vi "Test1_4.vi"() -> ()   [LabVIEW 2009]
uses:
  <instrlib>/Agilent 81150/Agilent 81150.lvlib
panel:
  in  "error in":errorcluster
  in  "Instrument VISA in":T1={"AWG VISA"="81160A", "Oscilloscope  VISA "="DSO80204B", "Integration Board IP"="172.16.7.43", "connection ID"=refnum}
  in  "Cycles Burst":i32=10000
  in  "DT_50_L0":i32[][](array[numeric])
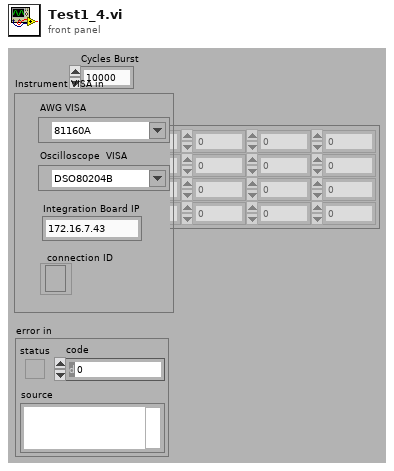
[diagram p1: front panel]
types:
  T1 = cluster{"AWG VISA":refnum<visa-resource-name>, "Oscilloscope  VISA ":refnum<visa-resource-name>, "Integration Board IP":string, "connection ID":refnum<k5>}
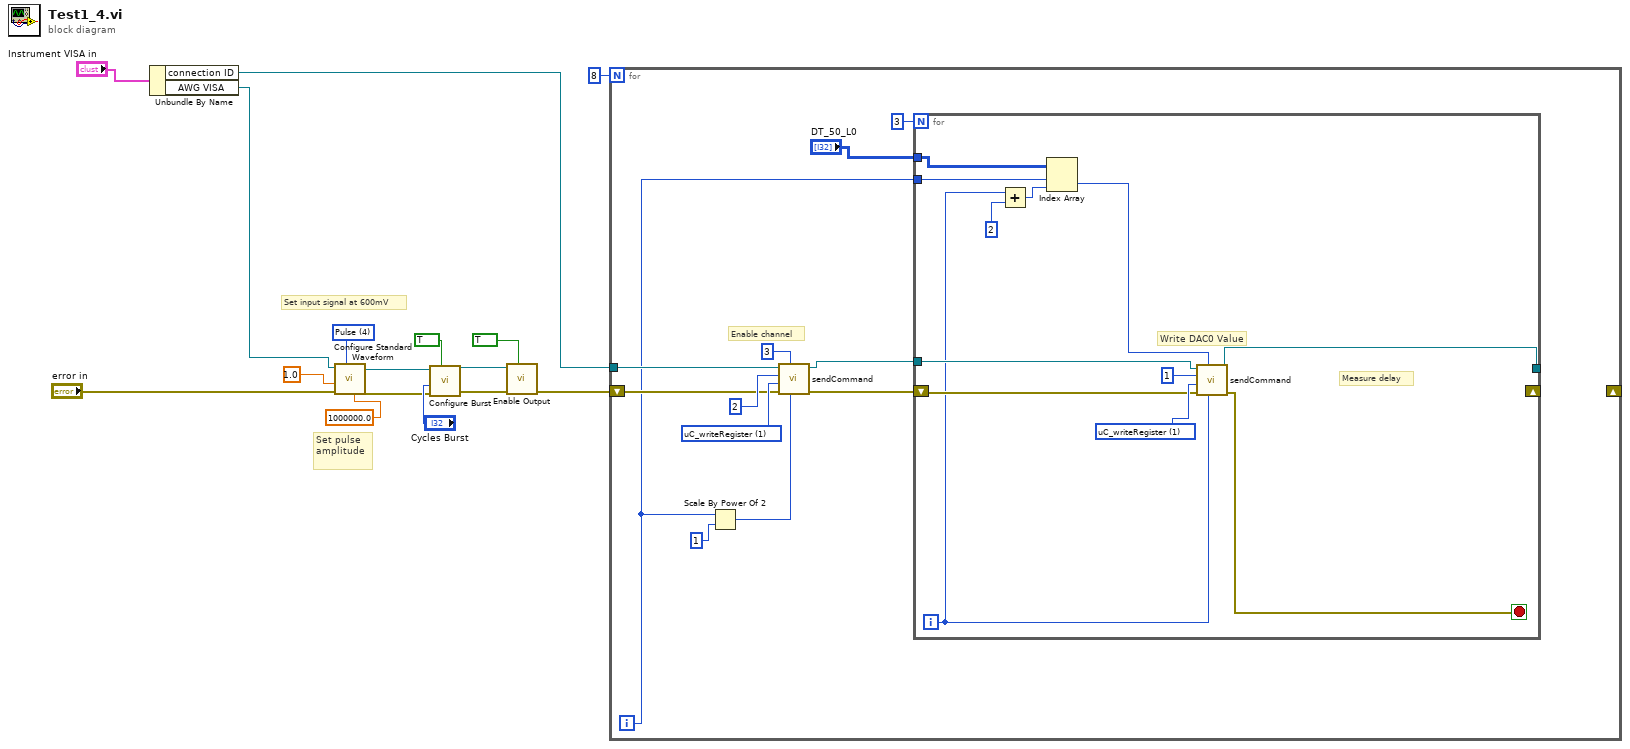
[diagram p0: block diagram]
diagram:
  w15 = u16 4 items=["Sine", "Square", "Ramp Up", "Ramp Down", "Pulse", "Noise", "DC"] ("Waveform (0: Sine)")
  # "Set input signal at 600mV"
  # "Set pulse amplitude"
  n1 = Unbundle By Name("Instrument VISA in") -> ("connection ID"=w3:refnum<k5>, "AWG VISA"=w1:refnum<visa-resource-name>)
  n2 = call <instrlib>:"Configure Standard Waveform.vi"("Frequency (1000.0 Hz)"=1000000.0, "Waveform (0: Sine)"=w15, "error in (no error)"="error in", "Amplitude (1.0 Vpp)"=1.0, "VISA resource name"=w1) -> ("error out"=w8:errorcluster, "VISA resource name out"=w7:refnum<visa-resource-name>)  [unwired: 5 in]
  n3 = call <instrlib>:"Configure Burst.vi"("Enable Burst (F: Disable)"=TRUE, "error in (no error)"=w8, "Burst Count (2)"="Cycles Burst", "VISA resource name"=w7) -> ("error out"=w11:errorcluster, "VISA resource name out"=w10:refnum<visa-resource-name>)  [unwired: 6 in]
  n4 = call <instrlib>:"Enable Output.vi"("Enable Output (T: Enable)"=TRUE, "error in (no error)"=w11, "VISA resource name"=w10) -> ("error out"=w2:errorcluster)  [unwired: 7 in, 1 out]
  n5 = for {
    N: 8 -> [_]
    tunnel: w3 -> [w20]
    shift-right: _ -> [_]
    shift-left: w2 -> [w19]
    i -> [w17]
    w26 = u16 1 items=["sendCommand"=9, "FPGA_writeRegister"=3, "FPGA_readRegister"=2, "uC_writeRegister"=1, "uC_readRegister"=0] ("Action")
    # "Enable channel"
    n6 = Scale By Power Of 2(n=w17, x=1) -> (x*2^n=w22:i32)
    n7 = call "sendCommand.vi"("Address"=w22, "Data"=3, "error in"=w19, "Action"=w26, "id_in"=2 ("id"), "connection ID"=w20) -> ("error out"=w21:errorcluster, "connection ID out"=w18:refnum<k5>)  [unwired: 1 in, 3 out]
    n8 = for {
      N: 3 -> [_]
      shift-right: _ -> [_]
      shift-left: w21 -> [w37]
      tunnel: "DT_50_L0" -> [w38]
      tunnel: [w35] -> _
      tunnel: w18 -> [w33]
      tunnel: w17 -> [w29]
      i -> [w30]
      stop <- w34 stop-if-true
      w40 = u16 1 items=["sendCommand"=9, "FPGA_writeRegister"=3, "FPGA_readRegister"=2, "uC_writeRegister"=1, "uC_readRegister"=0] ("Action")
      # "Measure delay"
      # "Write DAC0 Value"
      n9 = Add(x=w30, y=2 ("disabled index (col)")) -> (x+y=w31:i32)
      n10 = Index Array(array=w38, index (row)=w29, index (col)=w31) -> (element=w36:i32)
      n11 = call "sendCommand.vi"("Address"=w30, "Data"=w36, "error in"=w37, "Action"=w40, "id_in"=1 ("id"), "connection ID"=w33) -> ("error out"=w34:errorcluster, "connection ID out"=w35:refnum<k5>)  [unwired: 1 in, 3 out]
    }
  }
